vi "IsRunning.vi"(11 "status":u64) -> (3 "running?":bool)   [LabVIEW 2020, in "NI_TargetHelper.lvlib"]
uses:
  <vilib>/TargetSupport/NI_TargetHelper/NI_TargetHelper.lvlib
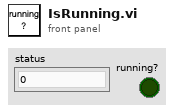
[diagram p1: front panel]
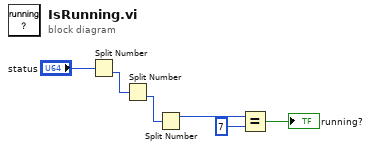
[diagram p0: block diagram]
diagram:
  n1 = Split Number(x="status") -> (lo(x)=w5:u32)  [unwired: 1 out]
  n2 = Split Number(x=w5) -> (lo(x)=w4:u16)  [unwired: 1 out]
  n3 = Split Number(x=w4) -> (hi(x)=w3:u8)  [unwired: 1 out]
  n4 = Equal?(x=w3, y=u8 7) -> (x = y?=→"running?":bool)
